vi "Save Theme.vi"(4 "input":T1={"Text.Font Name"="Segoe UI", "Text.Font Size"=30, "Color"=0, "Text.Justification"=enum."Center", "messge color"={"border"=14474460, "fill"=16777215}}, 6 "message font":T1={"Text.Font Name"="Segoe UI", "Text.Font Size"=30, "Color"=0, "Text.Justification"=enum."Center", "messge color"={"border"=16777215, "fill"=16777215}}, 8 "error in":errorcluster, 9 "button colors":T2={"false color"={"border"=14474460, "fill"=16777215}, "hover color"={"border"=14474460, "fill"=14474460}, "press color"={"border"=1067897, "fill"=1067897}, "Boolean Text"=1668818, "Text.Font Name"="", "Text.Font Size"=0, "Bold?"=TRUE, "Itallic?"=FALSE}, 10 "dialog colors":T3={"Header"=1668818, "Background"=1668818, "Picture Background"=16777216}, 11 "File":path=path "C:/Development/TSC.Pop-Up/tsc-default-theme.style") -> (0 "error out":errorcluster)   [LabVIEW 2021, in "Theme.lvclass"]
doc: "Save the theme data\n\n<b>Code Developed By:</b>\nTechnology Service Corporation\n1983 S Liberty Drive\nBloomington, IN 47403\nPhone: 812 558-7100\nwww.tsc.com/atcs\n\nDeveloper:\nDaniel Coons"
uses:
  Theme.lvclass
  Dialog colors--typedef.ctl
  Button colors--typedef.ctl
  message box--typdef.ctl
  Theme.lvclass/Theme.ctl
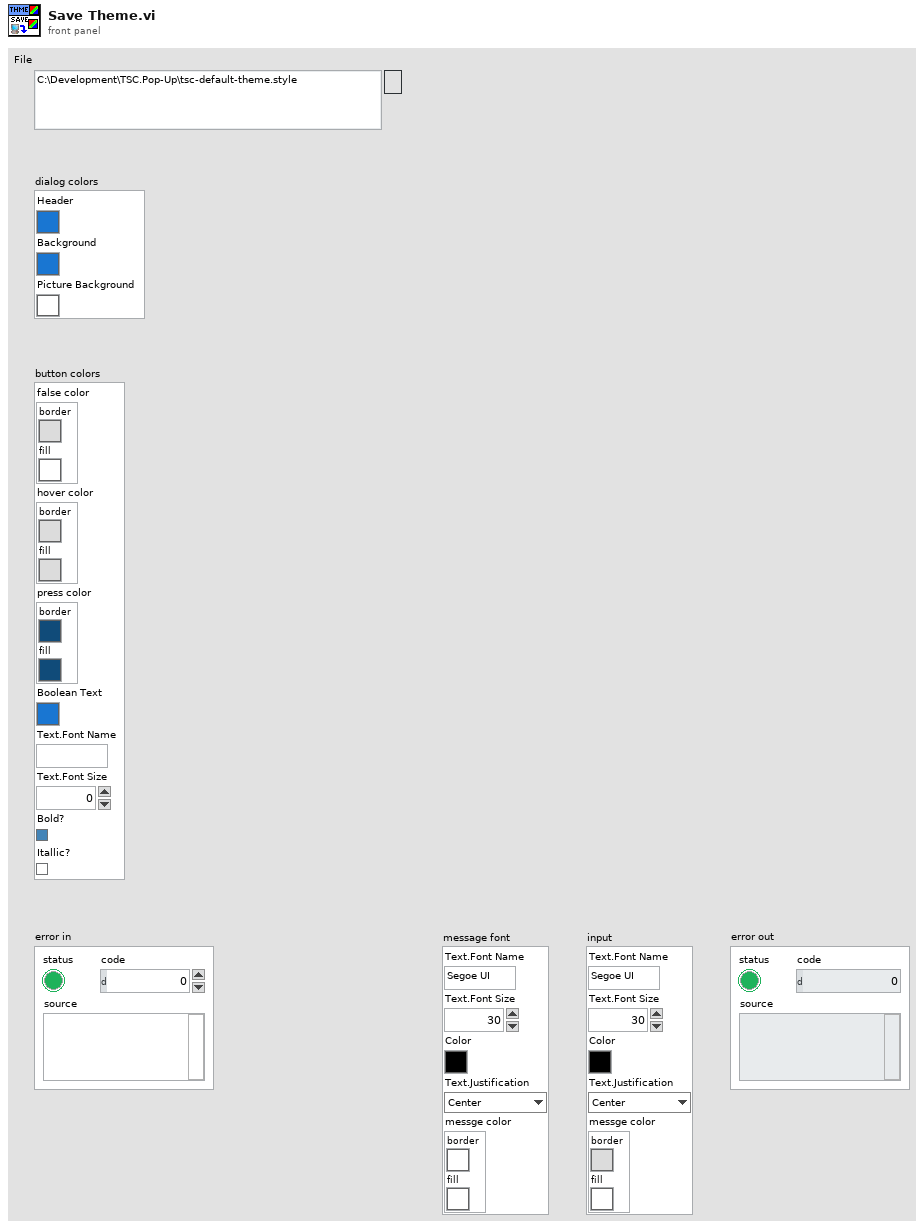
[diagram p1: front panel]
types:
  T1 = typedef "Theme.lvclass/message box--typdef.ctl" = cluster{"Text.Font Name":string, "Text.Font Size":u32, "Color":u32, "Text.Justification":enum16{"Left", "Center", "Right"}, "messge color":cluster{"border":u32, "fill":u32}}
  T2 = typedef "Theme.lvclass/Button colors--typedef.ctl" = cluster{"false color":cluster{"border":u32, "fill":u32}, "hover color":cluster{"border":u32, "fill":u32}, "press color":cluster{"border":u32, "fill":u32}, "Boolean Text":u32, "Text.Font Name":string, "Text.Font Size":u32, "Bold?":bool, "Itallic?":bool}
  T3 = typedef "Theme.lvclass/Dialog colors--typedef.ctl" = cluster{"Header":u32, "Background":u32, "Picture Background":u32}
  T4 = enum16{"open", "replace", "create", "open or create", "replace or create", "replace or create with confirmation"}
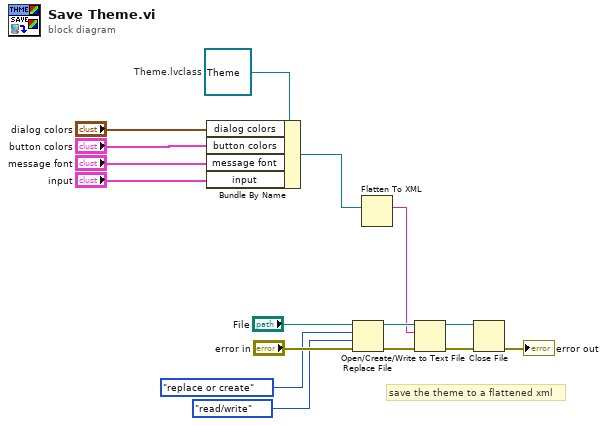
[diagram p0: block diagram]
diagram:
  w12 = refnum<class "Theme.lvclass"> refnum  # Theme.lvclass
  # "save the theme to a flattened xml"
  n1 = Bundle By Name(cluster=w12, "dialog colors"="dialog colors", "button colors"="button colors", "message font"="message font", "input"="input") -> (w2:refnum<class "Theme.lvclass">)
  n2 = Open/Create/Replace File(file path (use dialog)="File", error in="error in", operation (0:open)=T4."replace or create", access (0:read/write)=enum16{"read/write", "read-only", "write-only"}."read/write") -> (refnum out=w6:refnum<file>, error out=w15:errorcluster)  [unwired: 2 in, 1 out]
  n3 = Flatten To XML(6:w2) -> (2:w1:string)
  n4 = Write to Text File(file (use dialog)=w6, text=w1, error in=w15) -> (refnum out=w5:refnum<file>, error out=w13:errorcluster)  [unwired: 1 in, 1 out]
  n5 = Close File(refnum=w5, error in=w13) -> (error out=→"error out":errorcluster)  [unwired: 1 out]
